vi "Main.vi"() -> ()   [LabVIEW 2015]
doc: "Use this template to build a simple state machine design pattern. Each state executes code and determines which state to transition to."
uses:
  controls/State.ctl
  controls/Data.ctl
panel:
  out "Waveform Chart":dynamicdata(graph)
  in  "Do Something Else <Replace Me>":bool
  in  "Do Something":bool
  in  "Exit":bool
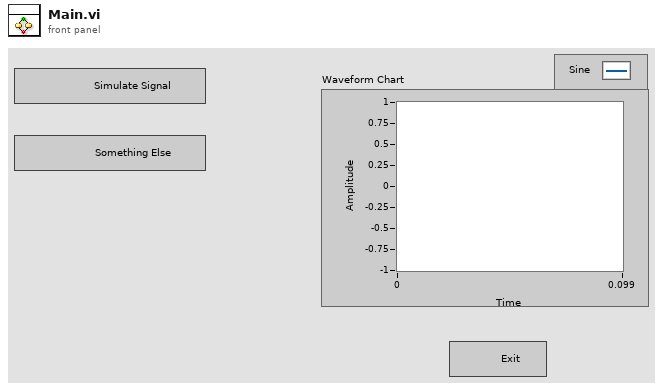
[diagram p1: front panel]
types:
  T1 = typedef "Data.ctl" = cluster{"Boolean <Replace Me>":bool, "String <Replace Me>":string, "Numeric <Replace Me>":dbl[]}
  T2 = typedef "State.ctl" = enum16{"Initialize", "Wait for Event", "String verknüpfen", "Messung simulieren", "User State 2", "Exit"}
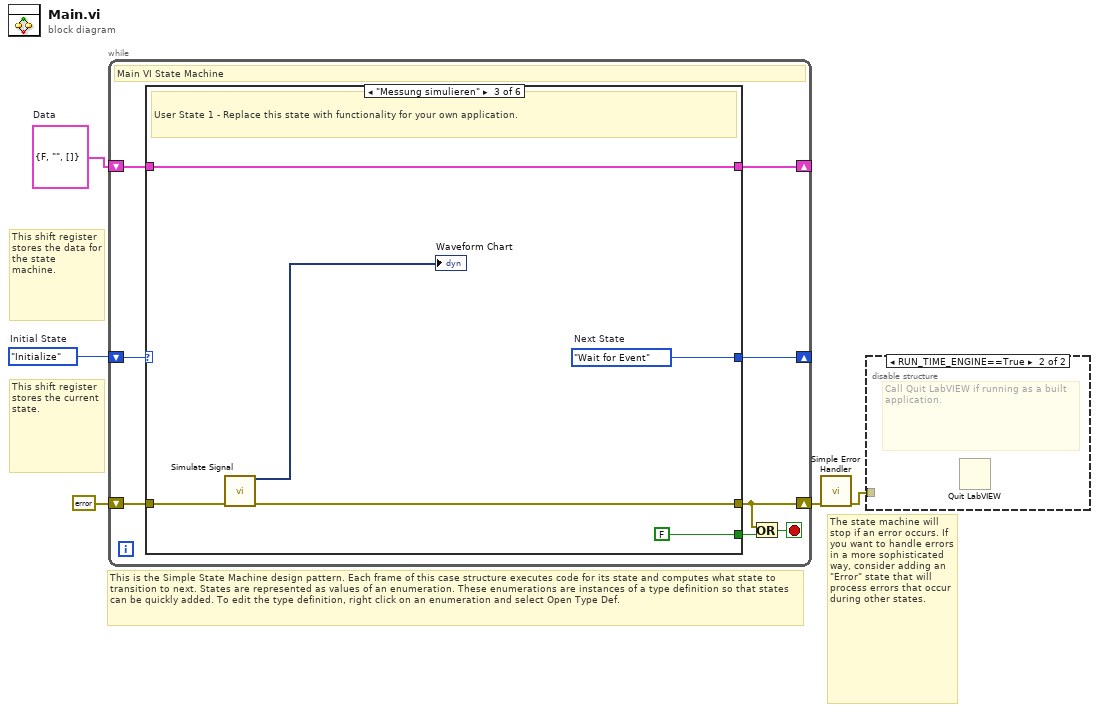
[diagram p0: block diagram]
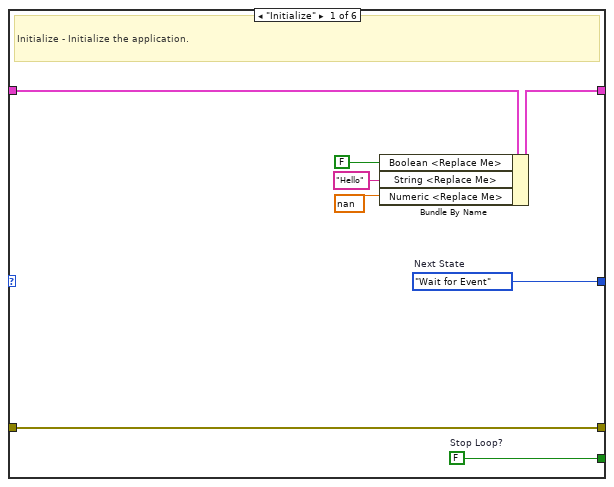
[diagram p3: hidden frame]
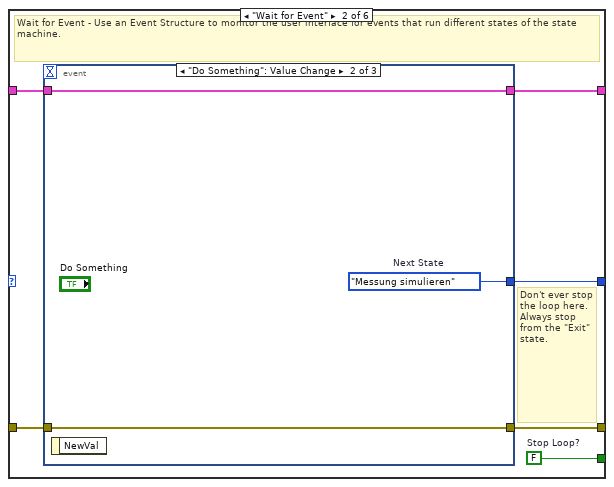
[diagram p4: hidden frame]
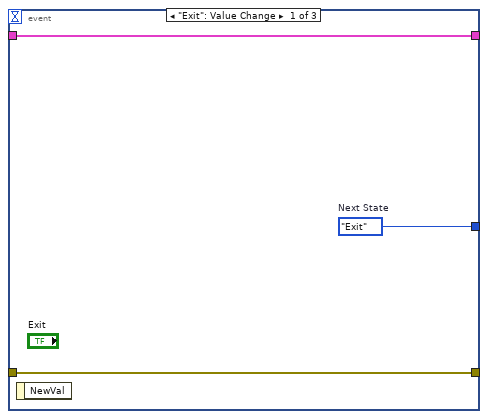
[diagram p5: hidden frame]
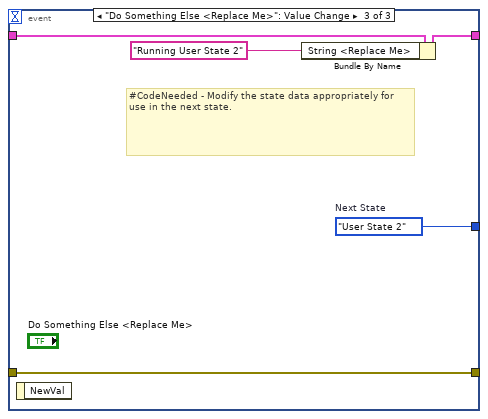
[diagram p6: hidden frame]
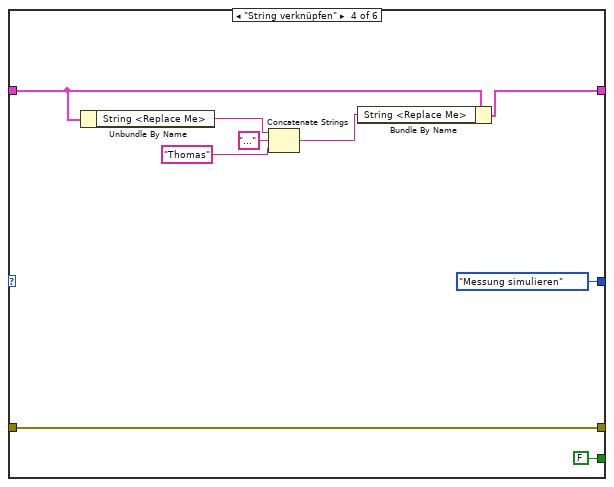
[diagram p7: hidden frame]
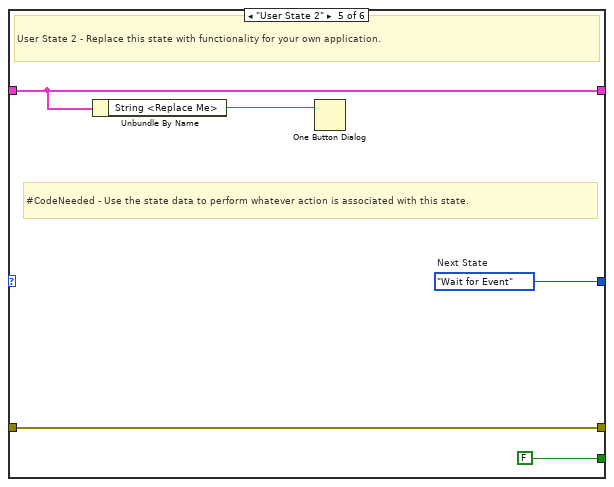
[diagram p8: hidden frame]
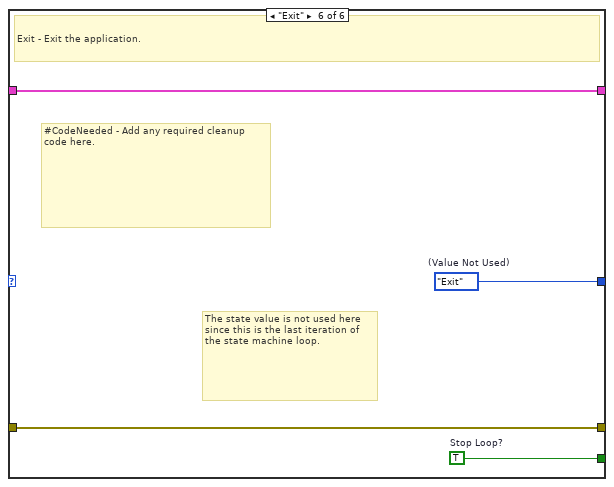
[diagram p9: hidden frame]
diagram:
  w4 = T1 {"Boolean <Replace Me>"=FALSE, "String <Replace Me>"="", "Numeric <Replace Me>"=[]}  # Data
  w5 = State."Initialize"  # Initial State
  # "The state machine will stop if an error occurs. If you want to handle errors in a more sophisticated way, consider adding an \"Error\" state that will process errors that occur during other states."
  # "This shift register stores the data for the state machine."
  # "This is the Simple State Machine design pattern. Each frame of this case structure executes code for its state and computes what state to transition to next. States are represented as values of an enumeration. These enumerations are instances of a type definition so that states can be quickly added. To edit the type definition, right click on an enumeration and select Open Type Def."
  # "This shift register stores the current state."
  n1 = while {
    shift-right: [w12] -> _
    shift-left: w5 -> [w13]
    shift-right: [w10] -> _
    shift-left: w4 -> [w11]
    shift-right: [w6] -> w2
    shift-left: errorcluster {"status"=FALSE, "code"=0, "source"=""} ("error constant") -> [w9]
    stop <- w7 stop-if-true
    # "Main VI State Machine"
    n2 = case shown="\"Messung simulieren\"" w13 {
      tunnel: [w21 w27 w44 State."Messung simulieren" ("(Value Not Used)") w58 w62] -> w12
      tunnel: [w20 w26 FALSE ("Stop Loop?") FALSE ("Stop Loop?") FALSE ("Stop Loop?") w60] -> w8
      tunnel: w11 -> [w19 w25 w42 w47 w56 w61]
      tunnel: [w18 w24 w42 w46 w56 w61] -> w10
      tunnel: w9 -> [w16 w23 w40 w53 w54 w59]
      tunnel: [w16 w22 w39 w53 w54 w59] -> w6
      frame "Initialize" {
        w20 = FALSE  # Stop Loop?
        w21 = State."Wait for Event"  # Next State
        # "Initialize - Initialize the application."
        n3 = Bundle By Name(cluster=w19, "Boolean <Replace Me>"=FALSE ("Replace_Me_Boolean"), "String <Replace Me>"="Hello", "Numeric <Replace Me>"=nan) -> (w18:T1)
      }
      frame "Wait for Event" {
        w26 = FALSE  # Stop Loop?
        # "Don't ever stop the loop here. Always stop from the \"Exit\" state."
        # "Wait for Event - Use an Event Structure to monitor the user interface for events that run different states of the state machine."
        n4 = event shown="[1] \"Do Something\": Value Change" {
          selector: _ -> [_ _ _]
          dyn-events: _ -> [_ _ _]
          timeout: _ -> [_ _ _]
          tunnel: [w30 w33 w38] -> w27
          tunnel: w25 -> [w29 w31 w37]
          tunnel: [w29 w31 w36] -> w24
          tunnel: w23 -> [w28 w32 w34]
          tunnel: [w28 w32 w34] -> w22
          event "Exit": Value Change {
            w30 = State."Exit"  # Next State
            n5 = event-data() -> ()  [unwired: 1 in, 1 out]
          }
          event "Do Something": Value Change {
            w33 = State."Messung simulieren"  # Next State
            n6 = event-data() -> ()  [unwired: 1 in, 1 out]
          }
          event "Do Something Else <Replace Me>": Value Change {
            w38 = State."User State 2"  # Next State
            # "#CodeNeeded - Modify the state data appropriately for use in the next state."
            n7 = event-data() -> ()  [unwired: 1 in, 1 out]
            n8 = Bundle By Name(cluster=w37, "String <Replace Me>"="Running User State 2" ("Running User State 2")) -> (w36:T1)
          }
        }
      }
      frame "Messung simulieren" {
        w44 = State."Wait for Event"  # Next State
        # "User State 1 - Replace this state with functionality for your own application."
        n9 = call "Simulate Signal"("error in (no error)"=w40) -> ("Sine"=→"Waveform Chart":dynamicdata, "error out"=w39:errorcluster)  [unwired: 13 in]
      }
      frame "String verknüpfen" {
        n10 = Unbundle By Name(w47) -> ("String <Replace Me>"=w50:string)
        n11 = Concatenate Strings(w50, "..." ("string"), "Thomas" ("string")) -> (w51:string)
        n12 = Bundle By Name(cluster=w47, "String <Replace Me>"=w51) -> (w46:T1)
      }
      frame "User State 2" {
        w58 = State."Wait for Event"  # Next State
        # "#CodeNeeded - Use the state data to perform whatever action is associated with this state."
        # "User State 2 - Replace this state with functionality for your own application."
        n13 = Unbundle By Name(w56) -> ("String <Replace Me>"=w55:string)
        n14 = One Button Dialog(message=w55) -> ()  [unwired: 1 in, 1 out]
      }
      frame "Exit" {
        w60 = TRUE  # Stop Loop?
        w62 = State."Exit"  # (Value Not Used)
        # "#CodeNeeded - Add any required cleanup code here."
        # "The state value is not used here since this is the last iteration of the state machine loop."
        # "Exit - Exit the application."
      }
    }
    n15 = Or(x=w6, y=w8) -> (x .or. y?=w7:bool)
  }
  n16 = call <vilib>:"Simple Error Handler.vi"("error in (no error)"=w2) -> ("error out"=w1:errorcluster)  [unwired: 4 in, 4 out]
  n17 = disable-structure shown="RUN_TIME_ENGINE==True" {
    disable-tunnel: w1 -> [_ _]
    frame condition #0 (active) {
    }
    frame condition #1 {
      # "Call Quit LabVIEW if running as a built application."
      n18 = Quit LabVIEW() -> ()  [unwired: 1 in]
    }
  }
